vi "Configure Temperature Setpoint.vi"(8 "error in (no error)":errorcluster, 10 "New Setpoint":dbl, 11 "heater_parent in":refnum<class "heater_parent.lvclass">) -> (0 "error out":errorcluster, 3 "heater_parent out":refnum<class "heater_parent.lvclass">)   [LabVIEW 2020, in "polar_bear_plus_drivers.lvlib" / "heater_parent.lvclass"]
doc: "Change the temperature setpoint."
uses:
  <instrlib>/RxnRover/Driver Polar Bear Plus/heater_parent/heater_parent.lvclass
  <instrlib>/RxnRover/Driver Polar Bear Plus/heater_parent/heater_parent.lvclass/heater_parent.ctl
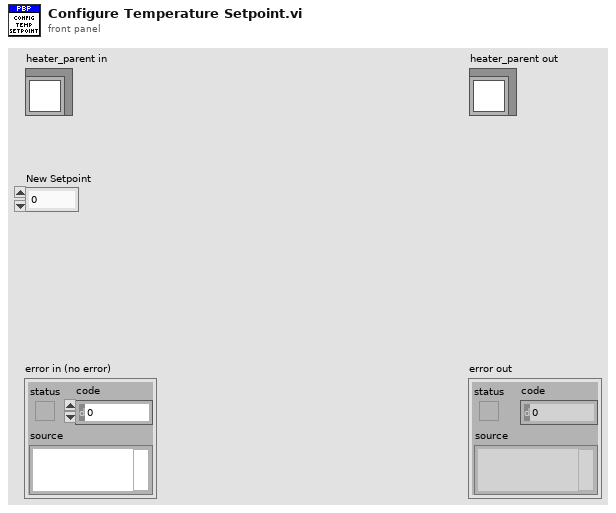
[diagram p1: front panel]
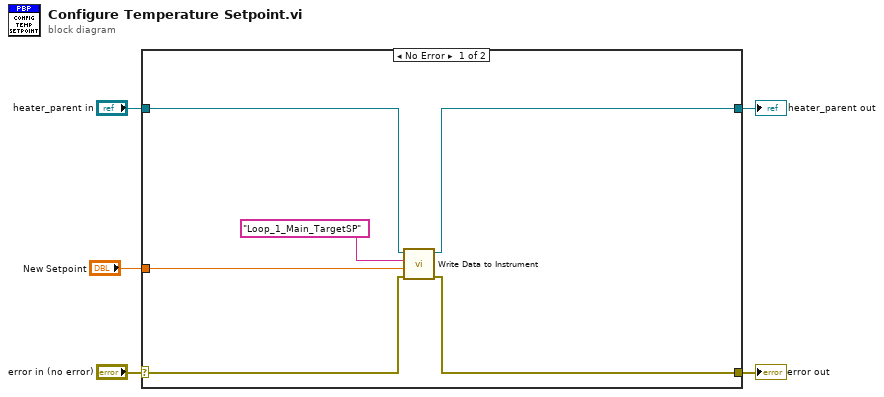
[diagram p0: block diagram]
diagram:
  n1 = case shown="No Error" "error in (no error)" {
    selector: "error in (no error)" -> [w10 w13]
    tunnel: [w9 w13] -> w4
    tunnel: [w8 w12] -> w2
    tunnel: "heater_parent in" -> [w11 w12]
    tunnel: "New Setpoint" -> [w7 _]
    frame No Error {
      n2 = call-dynamic "Write Data to Instrument.vi"("error in (no error)"=w10, "Value to Send"=w7, "Address"="Loop_1_Main_TargetSP", "heater_parent in"=w11) -> ("error out"=w9:errorcluster, "heater_parent out"=w8:refnum<class "heater_parent.lvclass">)  [unwired: 6 in]
    }
    frame Error {
    }
  }
  "error out" <- w4
  "heater_parent out" <- w2
